vi "Calculate prism values.vi"(7 "wavelength":dbl, 9 "c":dbl, 10 "b":dbl format="%#_13g", 11 "a":dbl) -> (3 "prism value":i32)   [LabVIEW 2017]
panel:
  out "Error out":errorcluster
  in  "Error in":errorcluster caption="Error in (no error)"
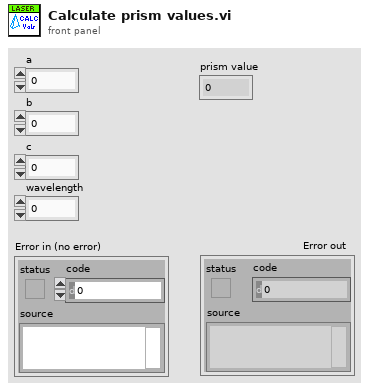
[diagram p1: front panel]
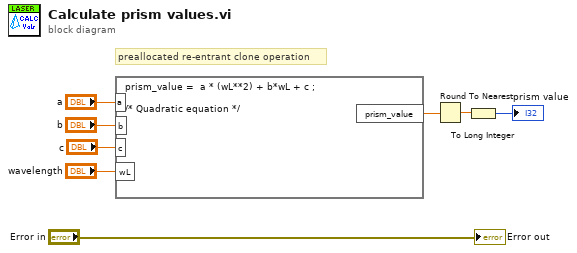
[diagram p0: block diagram]
diagram:
  # "preallocated re-entrant clone operation"
  n1 = formula code="prism_value =  a * (wL**2) + b*wL + c ;\n\n/* Quadratic equation */"("a"="a", "b"="b", "c"="c", "wL"="wavelength") -> ("prism_value"=w4:dbl)
  n2 = Round To Nearest(number=w4) -> (nearest integer value=w3:dbl)
  n3 = To Long Integer(number=w3) -> (32bit integer=→"prism value":i32)
  "Error out" <- "Error in"
